vi "Write ReadTimeout.vi"(8 "error in (no error)":errorcluster, 10 "ReadTimeout":i32=5000, 11 "Connection in":refnum<class "Connection.lvclass">) -> (0 "error out":errorcluster, 3 "Connection out":refnum<class "Connection.lvclass">)   [LabVIEW 2022 SP3, in "TcpSocket.lvlib" / "Connection.lvclass"]
uses:
  Connection.lvclass
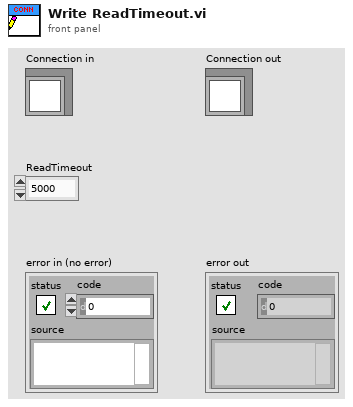
[diagram p1: front panel]
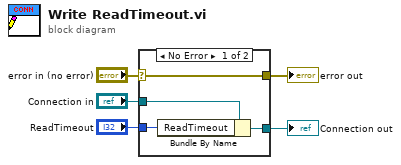
[diagram p0: block diagram]
diagram:
  n1 = case shown="No Error" "error in (no error)" {
    selector: "error in (no error)" -> [w9 w10]
    tunnel: [w9 w10] -> w4
    tunnel: [w7 w11] -> w2
    tunnel: "Connection in" -> [w8 w11]
    tunnel: "ReadTimeout" -> [w6 _]
    frame No Error {
      n2 = Bundle By Name(cluster=w8, "ReadTimeout"=w6) -> (w7:refnum<class "Connection.lvclass">)
    }
    frame Error {
    }
  }
  "error out" <- w4
  "Connection out" <- w2
